vi "All Frames Done.vi"(11 "Done in":bool) -> (3 "Done out":bool)   [LabVIEW 2015]
uses:
  <vilib>/rvi/Emulation/niFpgaSctlEmulationGetInTimedLoop.vi
  Globals/Global_Sample per Frame.vi
  <vilib>/rvi/Emulation/niFpgaProcessEmulError.vi
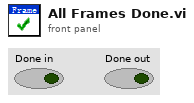
[diagram p1: front panel]
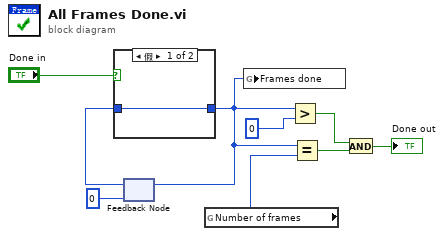
[diagram p0: block diagram]
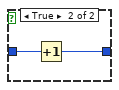
[diagram p2: hidden frame]
diagram:
  n1 = feedback #1(0) -> (w1:i32)
  n2 = case shown="假" "Done in" {
    tunnel: w1 -> [w10 w11]
    tunnel: [w10 w12] -> w4
    frame False {
    }
    frame True {
      n3 = Increment(x=w11) -> (x+1=w12:i32)
    }
  }
  n4 = feedback-in #1(w4) -> ()
  n5 = global read "Global_Sample per Frame.vi" "Number of frames"() -> (w3:i32)
  n6 = global write "Global_Sample per Frame.vi" "Frames done"(w4) -> ()
  n7 = Greater?(x=w4, y=0) -> (0:w6:bool)
  n8 = Equal?(x=w4, y=w3) -> (x = y?=w7:bool)
  n9 = And(x=w6, y=w7) -> (x .and. y?=→"Done out":bool)
